vi "Move.vi"(8 "error in (no error)":errorcluster, 9 "Y":dbl, 10 "X":dbl, 11 "VictorDrive in":refnum<class "VictorDrive.lvclass">) -> (0 "error out":errorcluster, 3 "VictorDrive out":refnum<class "VictorDrive.lvclass">)   [LabVIEW 2017, in "Drive.lvlib" / "VictorDrive.lvclass"]
uses:
  VictorDrive.lvclass
  VictorDrive.lvclass/VictorDrive.ctl
  <vilib>/Rock Robotics/SystemInterfaces/NetworkCommunication/NetComm_UsageReport_ResourceType.ctl
  Drive.lvclass
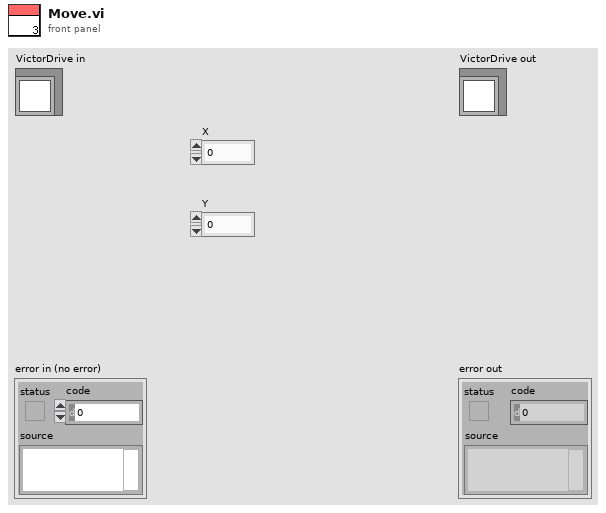
[diagram p1: front panel]
types:
  T1 = typedef "WPI_RobotDriveDevRef.ctl" = cluster{"DevStatus":errorcluster, "Motors[]":T2[], "Square Inputs":bool, "Max Output":dbl}
  T2 = typedef "WPI_MotorControlDeviceRef.ctl" = cluster{"DeviceStatus":errorcluster, "Type":T3, "PWM":cluster{"PWM Channel":T4, "DeadBand":T5}, "CAN":cluster{"Device Number":u8, "SetOutput VI Ref":variant, "GetOutput VI Ref":variant, "Enable VI Ref":variant, "Disable VI Ref":variant, "Data":variant}, "Invert":bool, "DIO PWM":cluster{"PWM \"Enable\" Channel":T4, "DIOChannel":T6, "PWM Rate":dbl}}
  T3 = typedef "WPI_MotorControlType.ctl" = enum16{"PWM", "CAN", "DIO PWM"}
  T4 = typedef "FPGA_DIOPWMChannel.ctl" = enum8{"PWM 0", "PWM 1", "PWM 2", "PWM 3", "PWM 4", "PWM 5", "PWM 6", "PWM 7", "PWM 8", "PWM 9", "PWM MXP 0", "PWM MXP 1", "PWM MXP 2", "PWM MXP 3", "PWM MXP 4", "PWM MXP 5", "PWM MXP 6", "PWM MXP 7", "PWM MXP 8", "PWM MXP 9", "Invalid"}
  T5 = typedef "WPI_PWMDeadband.ctl" = cluster{"Name":string, "maxPositivePwm":i32, "minPositivePwm":i32, "centerPwm":i32, "maxNegativePwm":i32, "minNegativePwm":i32, "angularRange":u16}
  T6 = typedef "FPGA_DIOChannel.ctl" = enum8{"DIO 0", "DIO 1", "DIO 2", "DIO 3", "DIO 4", "DIO 5", "DIO 6", "DIO 7", "DIO 8", "DIO 9", "DIO MXP 0", "DIO MXP 1", "DIO MXP 2", "DIO MXP 3", "DIO MXP 4", "DIO MXP 5", "DIO MXP 6", "DIO MXP 7", "DIO MXP 8", "DIO MXP 9", "DIO MXP 10", "DIO MXP 11", "DIO MXP 12", "DIO MXP 13", "DIO MXP 14", "DIO MXP 15", "SPI Port CS1", "SPI Port CS2", "SPI Port CS3", "SPI Port MISO", "SPI Port MOSI", "Invalid"}
  T7 = typedef "NetComm_UsageReport_ResourceType.ctl" = enum8{"Controller", "Module", "Language", "CANPlugin", "Accelerometer", "ADXL345", "AnalogChannel", "AnalogTrigger", "AnalogTriggerOutput", "CANJaguar", "Compressor", "Counter", "Dashboard", "DigitalInput", "DigitalOutput", "DriverStationCIO", "DriverStationEIO", "DriverStationLCD", "Encoder", "GearTooth", "Gyro", "I2C", "Framework", "Jaguar", "Joystick", "Kinect", "KinectStick", "PIDController", "Preferences", "PWM", "Relay", "RobotDrive", "SerialPort", "Servo", "Solenoid", "SPI", "Task", "Ultrasonic", "Victor", "Button", "Command", "AxisCamera", "PCVideoServer", "SmartDashboard", "Talon", "HiTechnicColorSensor", "HiTechnicAccel", "HiTechnicCompass", "SRF08", "AnalogOutput", "Victor SP", "Talon SRX", "CAN Talon SRX", "ADXL362 Accel", "ADXRS450 Gyro", "Rev SPARK", "Mindsensors SD540", "Digital Filter", "ADIS16448", "PDP", "PCM", "PigeonIMU", "Nidec Brushless", "CTRE CANifier", "CTRE Future 0", "CTRE Future 1", "CTRE Future 2", "CTRE Future 3", "CTRE Future 4", "CTRE Future 5", "CTRE Future 6"}
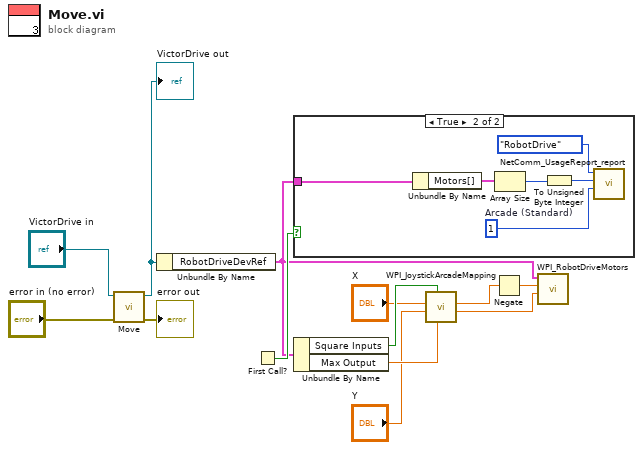
[diagram p0: block diagram]
diagram:
  n1 = call-parent "Move.vi"("error in (no error)"="error in (no error)", "Drive in"="VictorDrive in") -> ("error out"=→"error out":errorcluster, "Drive out"=w2:refnum<class "VictorDrive.lvclass">)  [unwired: 8 in]
  "VictorDrive out" <- w2
  n2 = Unbundle By Name(w2) -> ("RobotDriveDevRef"=w1:T1)
  n3 = First Call?() -> (First Call?: T/F=w10:bool)
  n4 = case shown="True" w10 {
    tunnel: w1 -> [_ w15]
    frame False {
    }
    frame True {
      w17 = u8 1  # Arcade (Standard)
      n5 = Unbundle By Name(w15) -> ("Motors[]"=w14:T2[])
      n6 = Array Size(array=w14) -> (size(s)=w16:i32)
      n7 = To Unsigned Byte Integer(number=w16) -> (unsigned 8bit integer=w18:u8)
      n8 = call <vilib>:"NetComm_UsageReport_report.vi"("Context"=w17, "Instance Number"=w18, "Resource Type"=NetComm_UsageReport_ResourceType."RobotDrive") -> ()  [unwired: 9 in]
    }
  }
  n9 = Unbundle By Name(w1) -> ("Square Inputs"=w9:bool, "Max Output"=w8:dbl)
  n10 = call <vilib>:"WPI_JoystickArcadeMapping.vi"("Max Output"=w8, "Square Inputs"=w9, "Y axis value"="Y", "X axis value"="X") -> ("Right Motor Value"=w7:dbl, "Left Motor Value"=w6:dbl)  [unwired: 6 in]
  n11 = Negate(x=w6) -> (-x=w5:dbl)
  n12 = call <vilib>:"WPI_RobotDriveMotors.vi"("RightSpeed"=w7, "LeftSpeed"=w5, "RobotDriveDevRef"=w1) -> ()  [unwired: 1 in, 8 out]
